vi "NMRFMTCP4.vi"() -> ()   [LabVIEW 2013]
uses:
  <vilib>/Analysis/2dsp.llb/Power Spectrum (DBL).vi
  kleinjan/MKS/Global - Pressure & Flow.vi
  <vilib>/Analysis/NI_AALBase.lvlib
  <vilib>/Analysis/NI_AALPro.lvlib
panel:
  out "Date / Time":string
  in  "Stop Run":bool=TRUE
  out "He readback":bool
  in  "Prompt?":bool
  out "He temp (K)":sgl=2.13326 format="%.3f"
  out "He press (torr)":sgl=33.89 format="%.3f"
  in  "NMR Channel Select":string(combo)="TEQ3560970472.csv"
  out "Color Box":u32(colorbox)=16775210
  out "Measurement":enum16{"TEQ", "POL", "QCV"}(ring)
  in  "IP Address":string="192.168.0.4"
  out "FFT Vrms":dbl[](graph)=[0.003860349127182048, 0.0026408786012199893, 0.0007110928431247576, 0.0002546953194851482, 0.00015606911370408223, 9.557131850537587e-05, 6.115097315115159e-05, 5.7012338680199956e-05, 3.020882234188072e-05, 4.4076193714080254e-05, 2.587519577753813e-05, 1.8713879048394136e-05, 1.6317240401098503e-05, 1.154265718789615e-05, 1.3123955910470731e-05, 1.3368904190798972e-05, 2.1885613497622673e-05, 1.798375515711528e-05, 4.375407331352679e-06, 8.732198758705414e-06, 2.6302534374244283e-06, 3.2949830538442704e-06, 1.1895815050496237e-05, 1.0182966066280883e-05, 1.8847898071173534e-06, 1.3934803392647094e-05, 1.052370134660737e-05, 1.3243501801509567e-05, 8.33538912191352e-06, 9.019609544923987e-06, 8.15332480790813e-06, 1.2373575068285524e-05, 6.708411703327406e-06, 6.22265423944835e-06, 5.068989993909897e-06, 3.0229813974287557e-06, 3.1089525018908967e-06, 5.953693945801889e-06, 6.206631518386126e-06, 6.229207375312059e-06, 4.1144781836691055e-06, 4.354798865838496e-06, 7.172496369868693e-06, 7.0098775910119696e-06, 2.191966447460206e-06, 1.5496079690644168e-06, 4.61696885546102e-06, 3.050901033352866e-06, 4.2174192750427694e-06, 7.930944150085501e-06, 6.689445166261909e-06, 2.1395244143303516e-06, 4.992797769241477e-06, 5.3745245406992406e-06, 6.062617096484538e-07, 8.270129726211426e-06, 3.5956569203627086e-06, 3.008894228477979e-06, 2.398514262112273e-06, 3.4988542677430917e-06, 1.4469323236866402e-06, 3.761661179538815e-06, 3.208518773411313e-06, 1.1187481039417038e-06, 5.7410915598327405e-06, 2.1784164294899814e-06, 3.898449684772871e-06, 3.52083007717426e-06, 1.9374004848225125e-06, 4.891889867434457e-06, 6.02715900907592e-06, 4.437968762435767e-06, 9.263245466394894e-07, 1.8616505810287503e-06, 5.23877964116065e-06, 3.0516904937122464e-06, 1.2800285909118407e-06, 3.507863659114302e-06, 6.239420652579072e-06, 5.998691457241049e-06, 5.312274179144818e-06, 3.3537794541369595e-06, 4.01592999534701e-06, 3.4824037830326406e-06, 3.0526271910251635e-06, 2.0097727604825172e-07, 4.607643528464001e-06, 5.424380631868744e-07, 4.160257383574649e-06, 2.972658642662555e-06, 1.9597322124373752e-06, 1.5255511381117527e-06, 2.103017178478501e-06, 5.198777606068562e-06, 2.9880903247162306e-06, 2.893406927495963e-06, 7.540072348828783e-06, 4.438692918242774e-06, 3.247269316126007e-06, 2.0747730164845625e-06, 6.856536235717e-06, 2.6481781470338664e-06, 3.0193029912273966e-06, 2.408089360787412e-06, 1.5854430464411955e-06, 1.8285871190437193e-06, 5.678656730464855e-06, 1.3784893037679748e-06, 4.116812883085481e-06, 4.819248986093936e-06, 4.5984658016483224e-06, 8.93008614072191e-06, 1.9094683248174202e-06, 9.416405140841326e-07, 5.047384071163484e-06, 3.197206859072784e-06, 1.794238609540721e-06, 3.313919423173037e-06, 2.714293243229963e-06, 3.535772500382675e-06, 3.499416768329835e-06, 4.63435639488753e-06, 5.034221148869452e-06, 1.8865455693025404e-06, 1.7901292369306268e-06, 4.424636665427706e-06, 5.615437490712334e-06, 2.466160580053458e-06, 2.1963153825552336e-06, 1.4846089900612258e-06, 4.302151200697518e-06, 5.254114798762438e-06, 3.1704642311621737e-06, 5.0703036462118136e-06, 1.354955104532314e-06, 3.0453363933660534e-06, 2.2463152825410145e-06, 3.808846738627808e-06, 3.7092372363585685e-06, 1.6325106978788555e-06, 3.2360511524404856e-06, 4.7480841852563215e-06, 5.2505859441000515e-06, 3.2850893327834457e-06, 1.934541747732607e-06, 3.029163168561454e-06, 1.9691995667214222e-06, 3.6405323264696174e-06, 5.056036709880387e-06, 1.919493519278465e-06, 5.595589965036569e-06, 1.852477214655658e-06, 2.8684687433525202e-06, 3.335542196883582e-06, 1.5704926166201195e-06, 3.7962328761918072e-06, 2.6584497284681668e-06, 3.4851642706109724e-06, 6.07788348181537e-06, 2.053548477567382e-06, 9.021564390261138e-07, 2.0277807693204723e-06, 4.32296683764549e-06, 4.064631037560265e-06, 3.8020871322129444e-06, 5.083401813415545e-06, 1.6733656079193586e-06, 1.745150362223994e-06, 8.979218241770401e-07, 1.531740077054345e-06, 5.921042959376128e-06, 2.424206120086413e-06, 6.426437182740756e-06, 5.5924058263776714e-06, 3.5215389749528754e-06, 8.300291245529953e-07, 4.411015274857682e-06, 2.563127166962874e-06, 5.846484935826142e-06, 3.130939375184453e-06, 2.719666304224687e-06, 7.360092224187938e-06, 1.7194250571999971e-06, 1.5443725434450432e-06, 3.822361300685473e-06, 3.923937068239552e-06, 2.89002198233437e-06, 1.614324549229591e-06, 2.999584927529115e-06, 2.060886472403204e-06, 1.3378034874859538e-06, 1.4706542842267576e-06, 3.536883042238073e-06, 7.249143652381299e-06, 1.267328794401466e-06, 1.1086696271129312e-06, 3.927146285844193e-06, 2.3360865908334468e-06, 2.672841677564323e-06, 3.4481594062109245e-06, 1.9525353575254287e-06, 1.9525353575254287e-06, 3.4481594062109245e-06, 2.672841677564323e-06, 2.3360865908334468e-06, 3.927146285844193e-06, 1.1086696271129312e-06, 1.267328794401466e-06, 7.249143652381299e-06, 3.536883042238073e-06, 1.4706542842267576e-06, 1.3378034874859538e-06, 2.060886472403204e-06, 2.999584927529115e-06, 1.614324549229591e-06, 2.89002198233437e-06, 3.923937068239552e-06, 3.822361300685473e-06, 1.5443725434450432e-06, 1.7194250571999971e-06, 7.360092224187938e-06, 2.719666304224687e-06, 3.130939375184453e-06, 5.846484935826142e-06, 2.563127166962874e-06, 4.411015274857682e-06, 8.300291245529953e-07, 3.5215389749528754e-06, 5.5924058263776714e-06, 6.426437182740756e-06, 2.424206120086413e-06, 5.921042959376128e-06, 1.531740077054345e-06, 8.979218241770401e-07, 1.745150362223994e-06, 1.6733656079193586e-06, 5.083401813415545e-06, 3.8020871322129444e-06, 4.064631037560265e-06, 4.32296683764549e-06, 2.0277807693204723e-06, 9.021564390261138e-07, 2.053548477567382e-06, 6.07788348181537e-06, 3.4851642706109724e-06, 2.6584497284681668e-06, 3.7962328761918072e-06, 1.5704926166201195e-06, 3.335542196883582e-06, 2.8684687433525202e-06, 1.852477214655658e-06, 5.595589965036569e-06, 1.919493519278465e-06, 5.056036709880387e-06, 3.6405323264696174e-06, 1.9691995667214222e-06, 3.029163168561454e-06, 1.934541747732607e-06, 3.2850893327834457e-06, 5.2505859441000515e-06, 4.7480841852563215e-06, 3.2360511524404856e-06, 1.6325106978788555e-06, 3.7092372363585685e-06, 3.808846738627808e-06, 2.2463152825410145e-06, 3.0453363933660534e-06, 1.354955104532314e-06, 5.0703036462118136e-06, 3.1704642311621737e-06, 5.254114798762438e-06, 4.302151200697518e-06, 1.4846089900612258e-06, 2.1963153825552336e-06, 2.466160580053458e-06, 5.615437490712334e-06, 4.424636665427706e-06, 1.7901292369306268e-06, 1.8865455693025404e-06, 5.034221148869452e-06, 4.63435639488753e-06, 3.499416768329835e-06, 3.535772500382675e-06, 2.714293243229963e-06, 3.313919423173037e-06, 1.794238609540721e-06, 3.197206859072784e-06, 5.047384071163484e-06, 9.416405140841326e-07, 1.9094683248174202e-06, 8.93008614072191e-06, 4.5984658016483224e-06, 4.819248986093936e-06, 4.116812883085481e-06, 1.3784893037679748e-06, 5.678656730464855e-06, 1.8285871190437193e-06, 1.5854430464411955e-06, 2.408089360787412e-06, 3.0193029912273966e-06, 2.6481781470338664e-06, 6.856536235717e-06, 2.0747730164845625e-06, 3.247269316126007e-06, 4.438692918242774e-06, 7.540072348828783e-06, 2.893406927495963e-06, 2.9880903247162306e-06, 5.198777606068562e-06, 2.103017178478501e-06, 1.5255511381117527e-06, 1.9597322124373752e-06, 2.972658642662555e-06, 4.160257383574649e-06, 5.424380631868744e-07, 4.607643528464001e-06, 2.0097727604825172e-07, 3.0526271910251635e-06, 3.4824037830326406e-06, 4.01592999534701e-06, 3.3537794541369595e-06, 5.312274179144818e-06, 5.998691457241049e-06, 6.239420652579072e-06, 3.507863659114302e-06, 1.2800285909118407e-06, 3.0516904937122464e-06, 5.23877964116065e-06, 1.8616505810287503e-06, 9.263245466394894e-07, 4.437968762435767e-06, 6.02715900907592e-06, 4.891889867434457e-06, 1.9374004848225125e-06, 3.52083007717426e-06, 3.898449684772871e-06, 2.1784164294899814e-06, 5.7410915598327405e-06, 1.1187481039417038e-06, 3.208518773411313e-06, 3.761661179538815e-06, 1.4469323236866402e-06, 3.4988542677430917e-06, 2.398514262112273e-06, 3.008894228477979e-06, 3.5956569203627086e-06, 8.270129726211426e-06, 6.062617096484538e-07, 5.3745245406992406e-06, 4.992797769241477e-06, 2.1395244143303516e-06, 6.689445166261909e-06, 7.930944150085501e-06, 4.2174192750427694e-06, 3.050901033352866e-06, 4.61696885546102e-06, 1.5496079690644168e-06, 2.191966447460206e-06, 7.0098775910119696e-06, 7.172496369868693e-06, 4.354798865838496e-06, 4.1144781836691055e-06, 6.229207375312059e-06, 6.206631518386126e-06, 5.953693945801889e-06, 3.1089525018908967e-06, 3.0229813974287557e-06, 5.068989993909897e-06, 6.22265423944835e-06, 6.708411703327406e-06, 1.2373575068285524e-05, 8.15332480790813e-06, 9.019609544923987e-06, 8.33538912191352e-06, 1.3243501801509567e-05, 1.052370134660737e-05, 1.3934803392647094e-05, 1.8847898071173534e-06, 1.0182966066280883e-05, 1.1895815050496237e-05, 3.2949830538442704e-06, 2.6302534374244283e-06, 8.732198758705414e-06, 4.375407331352679e-06, 1.798375515711528e-05, 2.1885613497622673e-05, 1.3368904190798972e-05, 1.3123955910470731e-05, 1.154265718789615e-05, 1.6317240401098503e-05, 1.8713879048394136e-05, 2.587519577753813e-05, 4.4076193714080254e-05, 3.020882234188072e-05, 5.7012338680199956e-05, 6.115097315115159e-05, 9.557131850537587e-05, 0.00015606911370408223, 0.0002546953194851482, 0.0007110928431247576, 0.0026408786012199893]
  out "Raw NMR Graph / Ave":cluster{dbl, "Step Width (MHz)":dbl, dbl[][]}(graph)={212.6, "Step Width (MHz)"=0.002, [[0.0121, 0.0117, 0.0117, 0.0117, 0.0114, 0.0113, 0.0113, 0.0111, 0.0111, 0.011, 0.011, 0.0108, 0.0107, 0.0105, 0.0105, 0.0104, 0.0099, 0.0099, 0.0098, 0.0096, 0.0096, 0.0095, 0.0095, 0.0093, 0.0093, 0.0092, 0.0089, 0.0089, 0.0087, 0.0085, 0.0084, 0.0084, 0.0081, 0.0081, 0.0079, 0.0079, 0.0078, 0.0076, 0.0076, 0.0076, 0.0075, 0.0073, 0.0073, 0.0072, 0.0072, 0.007, 0.0069, 0.0067, 0.0067, 0.0066, 0.0064, 0.0061, 0.0063, 0.0061, 0.006, 0.006, 0.0056, 0.0056, 0.0055, 0.0053, 0.0053, 0.0052, 0.0052, 0.005, 0.005, 0.0049, 0.0049, 0.0047, 0.0046, 0.0046, 0.0044, 0.0046, 0.0044, 0.0044, 0.0041, 0.0041, 0.004, 0.0038, 0.0038, 0.0038, 0.0035, 0.0035, 0.0035, 0.0034, 0.0034, 0.0034, 0.0032, 0.0031, 0.0029, 0.0029, 0.0029, 0.0029, 0.0027, 0.0026, 0.0026, 0.0026, 0.0024, 0.0024, 0.0023, 0.0021, 0.0021, 0.0021, 0.002, 0.002, 0.002, 0.0018, 0.0018, 0.0017, 0.0017, 0.0015, 0.0015, 0.0015, 0.0015, 0.0014, 0.0014, 0.0014, 0.0012, 0.0012, 0.0012, 0.0011, 0.0011, 0.0011, 0.0011, 0.0009, 0.0009, 0.0009, 0.0009, 0.0008, 0.0008, 0.0008, 0.0006, 0.0005, 0.0005, 0.0005, 0.0003, 0.0005, 0.0005, 0.0003, 0.0003, 0.0003, 0.0002, 0.0002, 0.0002, 0.0002, 0.0002, -0.0, -0.0, -0.0, -0.0, -0.0, -0.0, -0.0, -0.0, -0.0002, -0.0, -0.0, -0.0, -0.0002, -0.0, -0.0, -0.0, -0.0, -0.0, -0.0, -0.0, -0.0, -0.0, -0.0002, -0.0002, -0.0002, -0.0002, -0.0002, -0.0002, -0.0002, -0.0002, -0.0002, -0.0003, -0.0002, -0.0003, -0.0003, -0.0003, -0.0003, -0.0005, -0.0003, -0.0003, -0.0003, -0.0003, -0.0003, -0.0003, -0.0003, -0.0003, -0.0003, -0.0003, -0.0003, -0.0005, -0.0003, -0.0005, -0.0005, -0.0006, -0.0003, -0.0003, -0.0003, -0.0003, -0.0003, -0.0003, -0.0003, -0.0002, -0.0003, -0.0003, -0.0003, -0.0002, -0.0003, -0.0002, -0.0002, -0.0002, -0.0, -0.0, -0.0, -0.0002, -0.0002, -0.0, -0.0, -0.0, -0.0, -0.0, -0.0, -0.0, -0.0, -0.0, -0.0, -0.0, -0.0, -0.0, -0.0, -0.0, 0.0002, -0.0, 0.0002, -0.0, 0.0002, 0.0002, 0.0003, 0.0002, 0.0002, 0.0003, 0.0003, 0.0005, 0.0003, 0.0005, 0.0005, 0.0005, 0.0006, 0.0006, 0.0008, 0.0008, 0.0009, 0.0008, 0.0008, 0.0009, 0.0008, 0.0009, 0.0009, 0.0008, 0.0011, 0.0009, 0.0011, 0.0012, 0.0012, 0.0014, 0.0014, 0.0014, 0.0015, 0.0015, 0.0015, 0.0017, 0.0017, 0.0017, 0.0018, 0.0018, 0.0018, 0.0018, 0.0018, 0.0018, 0.002, 0.002, 0.0021, 0.0023, 0.0023, 0.0023, 0.0023, 0.0024, 0.0026, 0.0026, 0.0027, 0.0027, 0.0029, 0.0029, 0.0029, 0.0031, 0.0031, 0.0031, 0.0031, 0.0034, 0.0034, 0.0035, 0.0035, 0.0035, 0.0037, 0.0037, 0.0038, 0.0038, 0.0038, 0.004, 0.004, 0.0041, 0.0041, 0.0043, 0.0044, 0.0044, 0.0046, 0.0047, 0.0047, 0.0049, 0.0049, 0.0052, 0.0052, 0.005, 0.0052, 0.0053, 0.0053, 0.0055, 0.0055, 0.0058, 0.0058, 0.0058, 0.0058, 0.006, 0.0061, 0.0061, 0.0063, 0.0064, 0.0066, 0.0066, 0.0066, 0.0067, 0.0069, 0.007, 0.0072, 0.0072, 0.0073, 0.0075, 0.0075, 0.0076, 0.0076, 0.0078, 0.0078, 0.0079, 0.0081, 0.0082, 0.0084, 0.0084, 0.0085, 0.0085, 0.0087, 0.0089, 0.0089, 0.0089, 0.0092, 0.0093, 0.0093, 0.0095, 0.0096, 0.0096, 0.0096, 0.0099, 0.0099, 0.0101, 0.0101, 0.0102, 0.0104, 0.0105, 0.0105, 0.0107, 0.0108, 0.011, 0.011, 0.011, 0.0111, 0.0113, 0.0114, 0.0116, 0.0116, 0.0117, 0.0119, 0.0119, 0.0121, 0.0122, 0.0124, 0.0125, 0.0125, 0.0127], [0.0, 0.0, 0.0, 0.0, 0.0, 0.0, 0.0, 0.0, 0.0, 0.0, 0.0, 0.0, 0.0, 0.0, 0.0, 0.0, 0.0, 0.0, 0.0, 0.0, 0.0, 0.0, 0.0, 0.0, 0.0, 0.0, 0.0, 0.0, 0.0, 0.0, 0.0, 0.0, 0.0, 0.0, 0.0, 0.0, 0.0, 0.0, 0.0, 0.0, 0.0, 0.0, 0.0, 0.0, 0.0, 0.0, 0.0, 0.0, 0.0, 0.0, 0.0, 0.0, 0.0, 0.0, 0.0, 0.0, 0.0, 0.0, 0.0, 0.0, 0.0, 0.0, 0.0, 0.0, 0.0, 0.0, 0.0, 0.0, 0.0, 0.0, 0.0, 0.0, 0.0, 0.0, 0.0, 0.0, 0.0, 0.0, 0.0, 0.0, 0.0, 0.0, 0.0, 0.0, 0.0, 0.0, 0.0, 0.0, 0.0, 0.0, 0.0, 0.0, 0.0, 0.0, 0.0, 0.0, 0.0, 0.0, 0.0, 0.0, 0.0, 0.0, 0.0, 0.0, 0.0, 0.0, 0.0, 0.0, 0.0, 0.0, 0.0, 0.0, 0.0, 0.0, 0.0, 0.0, 0.0, 0.0, 0.0, 0.0, 0.0, 0.0, 0.0, 0.0, 0.0, 0.0, 0.0, 0.0, 0.0, 0.0, 0.0, 0.0, 0.0, 0.0, 0.0, 0.0, 0.0, 0.0, 0.0, 0.0, 0.0, 0.0, 0.0, 0.0, 0.0, 0.0, 0.0, 0.0, 0.0, 0.0, 0.0, 0.0, 0.0, 0.0, 0.0, 0.0, 0.0, 0.0, 0.0, 0.0, 0.0, 0.0, 0.0, 0.0, 0.0, 0.0, 0.0, 0.0, 0.0, 0.0, 0.0, 0.0, 0.0, 0.0, 0.0, 0.0, 0.0, 0.0, 0.0, 0.0, 0.0, 0.0, 0.0, 0.0, 0.0, 0.0, 0.0, 0.0, 0.0, 0.0, 0.0, 0.0, 0.0, 0.0, 0.0, 0.0, 0.0, 0.0, 0.0, 0.0, 0.0, 0.0, 0.0, 0.0, 0.0, 0.0, 0.0, 0.0, 0.0, 0.0, 0.0, 0.0, 0.0, 0.0, 0.0, 0.0, 0.0, 0.0, 0.0, 0.0, 0.0, 0.0, 0.0, 0.0, 0.0, 0.0, 0.0, 0.0, 0.0, 0.0, 0.0, 0.0, 0.0, 0.0, 0.0, 0.0, 0.0, 0.0, 0.0, 0.0, 0.0, 0.0, 0.0, 0.0, 0.0, 0.0, 0.0, 0.0, 0.0, 0.0, 0.0, 0.0, 0.0, 0.0, 0.0, 0.0, 0.0, 0.0, 0.0, 0.0, 0.0, 0.0, 0.0, 0.0, 0.0, 0.0, 0.0, 0.0, 0.0, 0.0, 0.0, 0.0, 0.0, 0.0, 0.0, 0.0, 0.0, 0.0, 0.0, 0.0, 0.0, 0.0, 0.0, 0.0, 0.0, 0.0, 0.0, 0.0, 0.0, 0.0, 0.0, 0.0, 0.0, 0.0, 0.0, 0.0, 0.0, 0.0, 0.0, 0.0, 0.0, 0.0, 0.0, 0.0, 0.0, 0.0, 0.0, 0.0, 0.0, 0.0, 0.0, 0.0, 0.0, 0.0, 0.0, 0.0, 0.0, 0.0, 0.0, 0.0, 0.0, 0.0, 0.0, 0.0, 0.0, 0.0, 0.0, 0.0, 0.0, 0.0, 0.0, 0.0, 0.0, 0.0, 0.0, 0.0, 0.0, 0.0, 0.0, 0.0, 0.0, 0.0, 0.0, 0.0, 0.0, 0.0, 0.0, 0.0, 0.0, 0.0, 0.0, 0.0, 0.0, 0.0, 0.0, 0.0, 0.0, 0.0, 0.0, 0.0, 0.0, 0.0, 0.0, 0.0, 0.0, 0.0, 0.0, 0.0, 0.0, 0.0, 0.0, 0.0, 0.0, 0.0, 0.0, 0.0, 0.0, 0.0, 0.0, 0.0, 0.0, 0.0, 0.0, 0.0, 0.0, 0.0, 0.0, 0.0, 0.0, 0.0, 0.0, 0.0, 0.0, 0.0, 0.0, 0.0, 0.0, 0.0, 0.0, 0.0, 0.0]]}
  in  "GPIB Addr (28)":refnum<visa-resource-name>="GPIB1::28::INSTR"
  out "Pedestal (V)":dbl=0.006282083333333333 format="%_2g"
  in  "Open Global Panel":bool=TRUE
  out "Peak center (MHz)":sgl=213.38817 format="%.3f"
  out "Telnet error out":errorcluster
  out "+3.3V supply":dbl=3.265 format="%_4g"
  out "Temp (C)":dbl=27.5 format="%_4g"
  out "RF OK":bool=TRUE
  out "Peak area (V-MHz)":sgl=-1.9332666 format="%.5f"
  out "# Good Spectra":i32=1000
  out "Pedestal OK":bool=TRUE
  out "Sweep #":i32=6
  out "1st Sweep":bool
  out "ADC volts OK":bool=TRUE
  out "Peak Height Distribution":cluster{"Y":dbl[], "Y":dbl[]}[](graph)=[{"Y"=[0.008008147916666668, 0.008026943750000001, 0.008045739583333334, 0.008064535416666668, 0.00808333125, 0.008102127083333334, 0.008120922916666667, 0.00813971875, 0.008158514583333333, 0.008177310416666667, 0.00819610625, 0.008214902083333335, 0.008233697916666668, 0.008252493750000001, 0.008271289583333334, 0.008290085416666667, 0.00830888125, 0.008327677083333334, 0.008346472916666667, 0.00836526875, 0.008384064583333333, 0.008402860416666666, 0.008421656250000001, 0.008440452083333334, 0.008459247916666668, 0.00847804375, 0.008496839583333334, 0.008515635416666667, 0.00853443125, 0.008553227083333333, 0.008572022916666667, 0.00859081875, 0.008609614583333333, 0.008628410416666668, 0.008647206250000001, 0.008666002083333334, 0.008684797916666667, 0.00870359375, 0.008722389583333334, 0.008741185416666667, 0.00875998125, 0.008778777083333333, 0.008797572916666666, 0.00881636875, 0.008835164583333333, 0.008853960416666667, 0.00887275625, 0.008891552083333334, 0.008910347916666667, 0.00892914375, 0.008947939583333333, 0.008966735416666666, 0.00898553125, 0.009004327083333333, 0.009023122916666666, 0.009041918749999999, 0.009060714583333334, 0.009079510416666667, 0.00909830625, 0.009117102083333333, 0.009135897916666667, 0.00915469375, 0.009173489583333333, 0.009192285416666666, 0.00921108125, 0.009229877083333332, 0.009248672916666666, 0.00926746875, 0.009286264583333334, 0.009305060416666667, 0.00932385625, 0.009342652083333333, 0.009361447916666666, 0.00938024375, 0.009399039583333333, 0.009417835416666666, 0.009436631249999999, 0.009455427083333332, 0.009474222916666667, 0.00949301875, 0.009511814583333333, 0.009530610416666667, 0.00954940625, 0.009568202083333333, 0.009586997916666666, 0.00960579375, 0.009624589583333332, 0.009643385416666666, 0.009662181249999999, 0.009680977083333334, 0.009699772916666667, 0.00971856875, 0.009737364583333333, 0.009756160416666666, 0.00977495625, 0.009793752083333333, 0.009812547916666666, 0.009831343749999999, 0.009850139583333332, 0.009868935416666665], "Y"=[1.0, 0.0, 0.0, 1.0, 1.0, 0.0, 2.0, 1.0, 1.0, 1.0, 2.0, 2.0, 4.0, 2.0, 2.0, 3.0, 3.0, 3.0, 4.0, 3.0, 5.0, 6.0, 4.0, 4.0, 7.0, 3.0, 10.0, 5.0, 10.0, 7.0, 9.0, 8.0, 14.0, 12.0, 9.0, 16.0, 10.0, 17.0, 13.0, 14.0, 12.0, 10.0, 24.0, 21.0, 12.0, 18.0, 16.0, 23.0, 22.0, 15.0, 16.0, 19.0, 16.0, 19.0, 14.0, 17.0, 23.0, 22.0, 22.0, 24.0, 23.0, 22.0, 17.0, 25.0, 18.0, 23.0, 20.0, 14.0, 14.0, 10.0, 18.0, 20.0, 10.0, 20.0, 16.0, 10.0, 13.0, 14.0, 12.0, 11.0, 15.0, 10.0, 11.0, 7.0, 6.0, 9.0, 0.0, 8.0, 3.0, 3.0, 4.0, 3.0, 3.0, 1.0, 0.0, 0.0, 0.0, 1.0, 1.0, 1.0]}]
  out "S/N":dbl=26.093843753781734 format="%_3g"
  out "Peak mean (V)":dbl=0.009030414166666665 format="%_4g"
  out "Pedestal Diff (V)":sgl=0.0009175 format="%.3f"
  out "Peak amp (V)":sgl=0.0064179166 format="%.3f"
  out "SMT error out":errorcluster
  out "Peak RMS (mV)":dbl=0.3460745090633841 format="%.3f"
  # "E1039 NMR Panel"
  # "Results"
  # "A\nv\ne\nr\na\ng\ne\ns"
  # "S\nw\ne\ne\np"
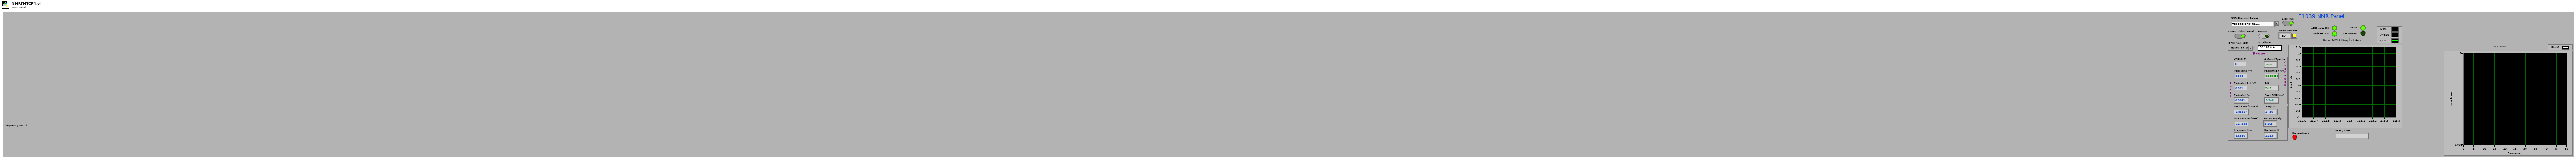
[diagram p1: front panel]
types:
  T1 = enum32{"Invalid", "Standard", "Closed", "Hidden", "Minimized", "Maximized"}
  T2 = enum32{"Bad", "Idle", "Run top level", "Running"}
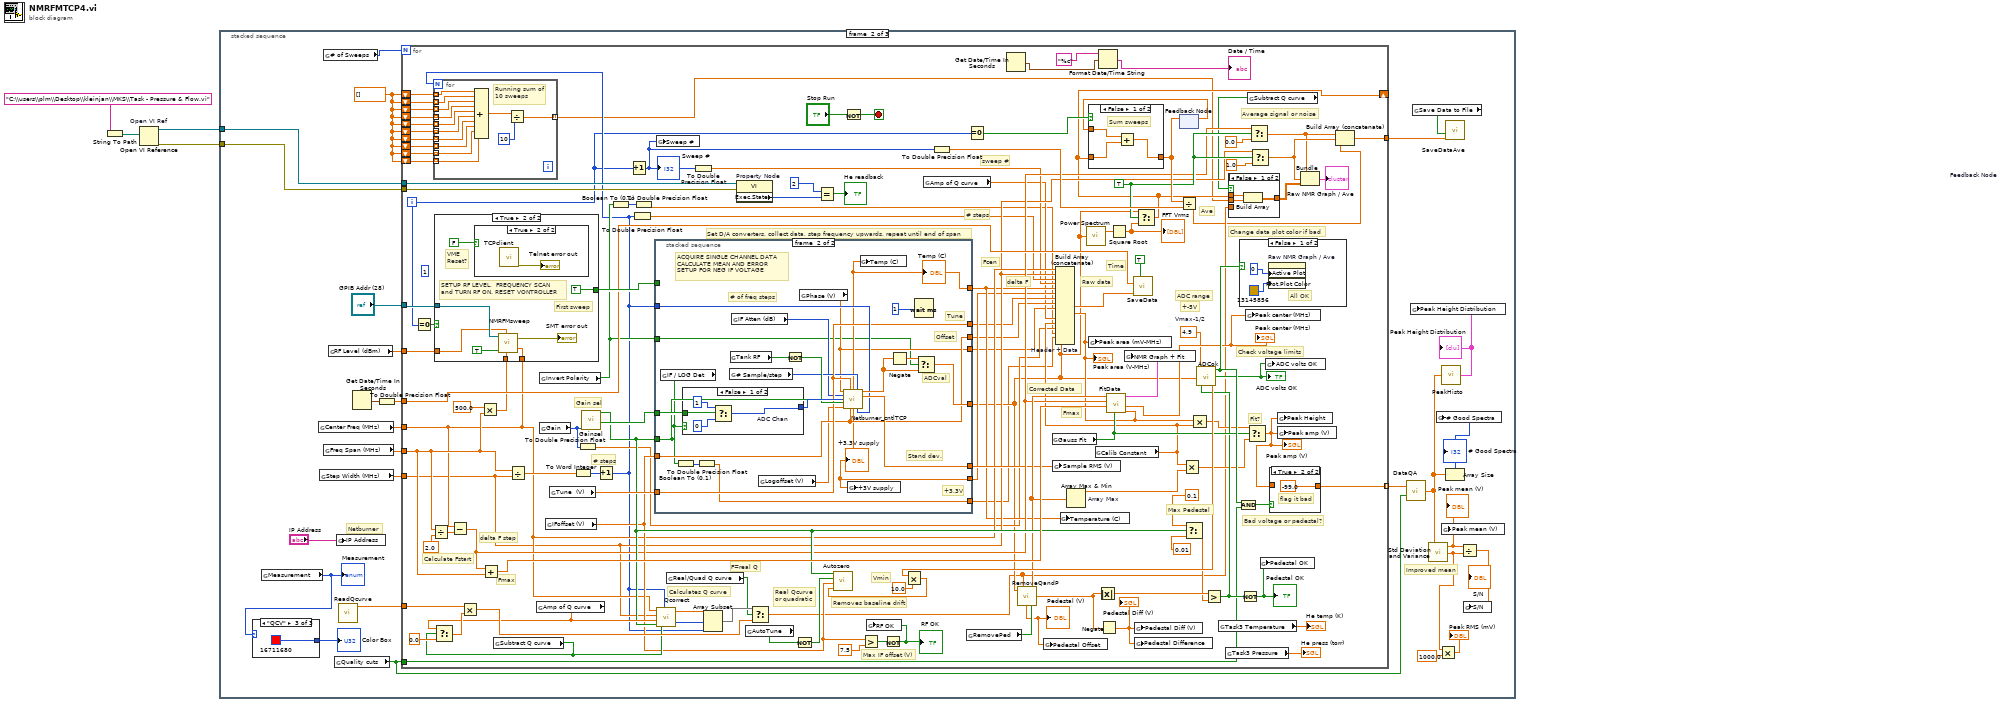
[diagram p0: block diagram]
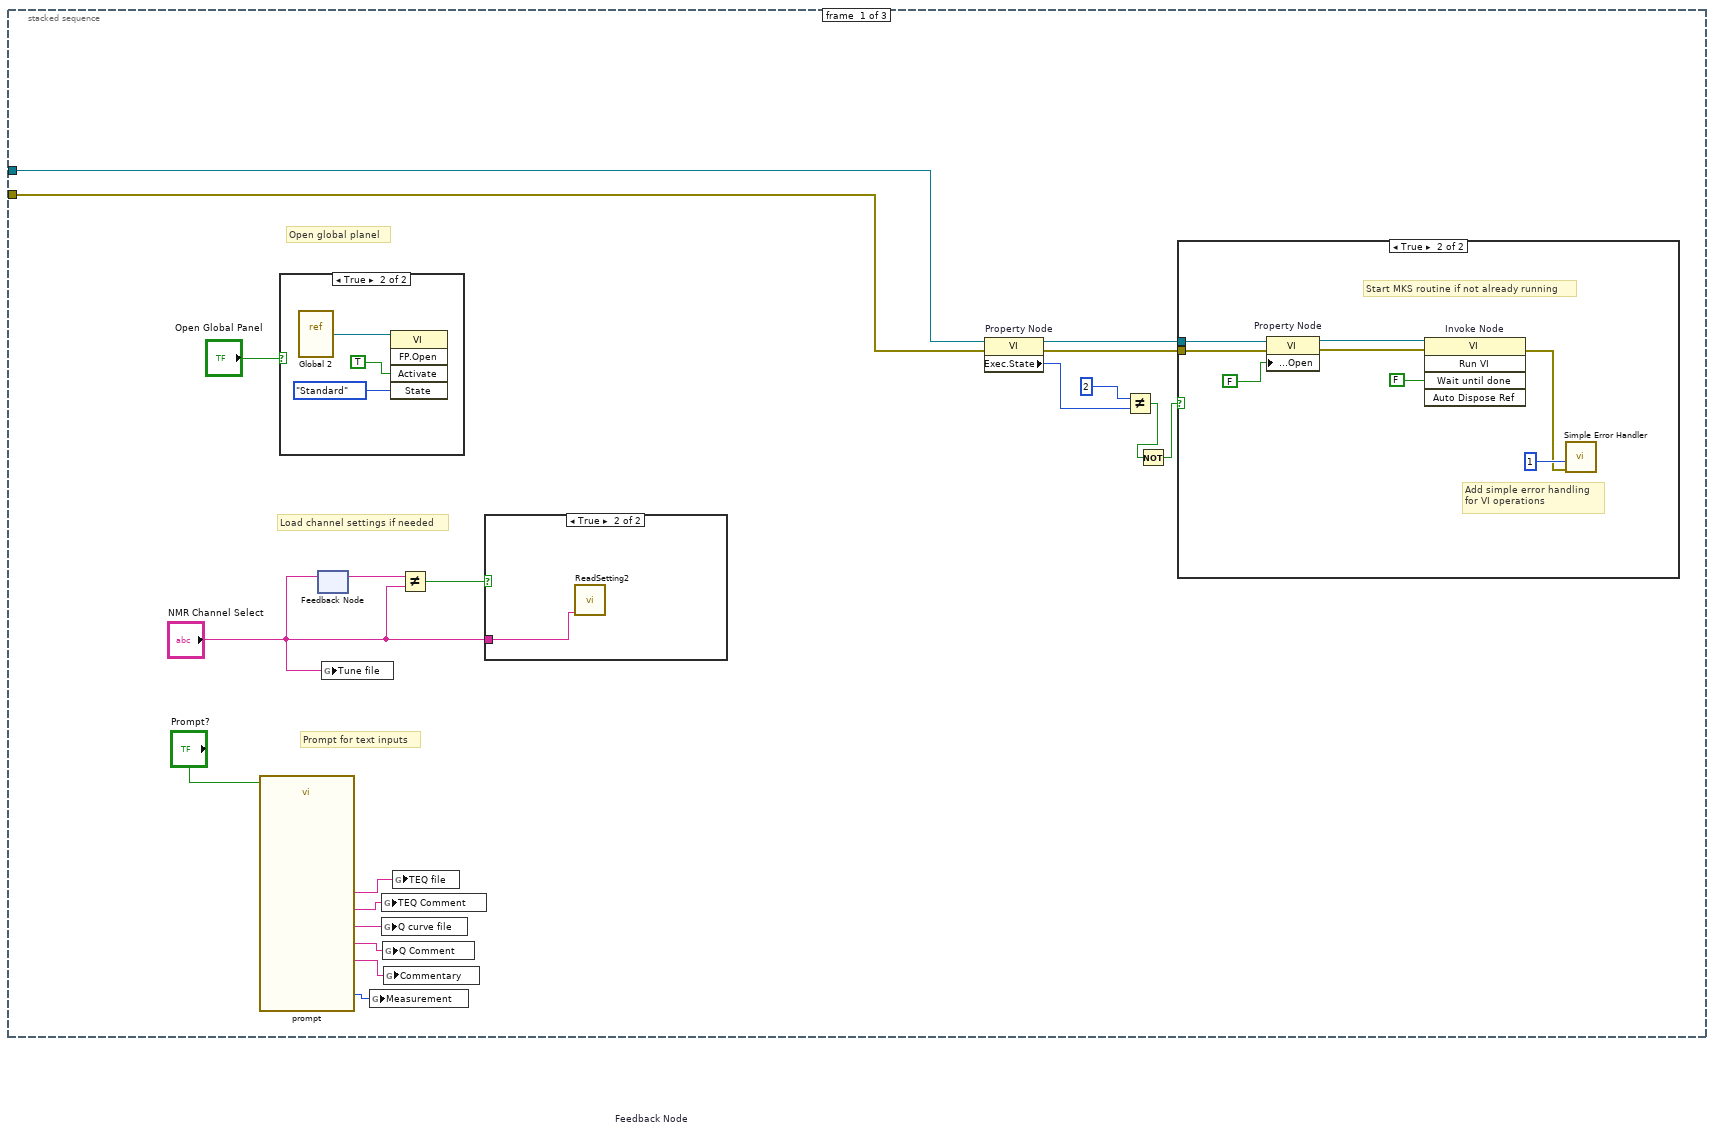
[diagram p2: hidden frame]
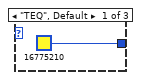
[diagram p6: hidden frame]
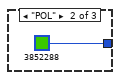
[diagram p7: hidden frame]
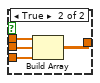
[diagram p8: hidden frame]
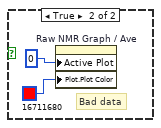
[diagram p10: hidden frame]
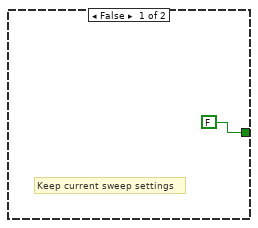
[diagram p12: hidden frame]
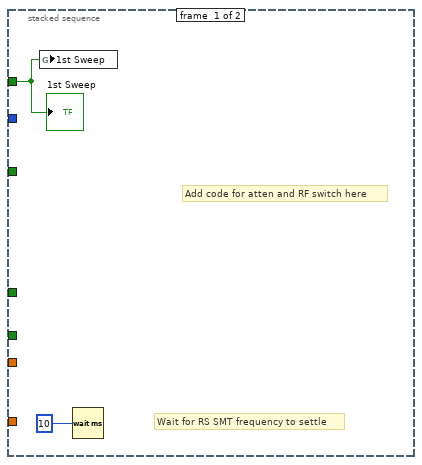
[diagram p14: hidden frame]
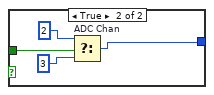
[diagram p15: hidden frame]
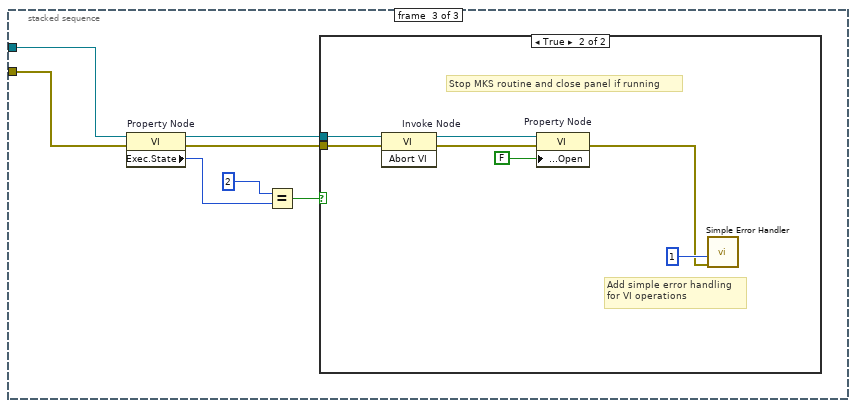
[diagram p16: hidden frame]
diagram:
  n1 = String To Path(string="C:\\users\\plm\\Desktop\\kleinjan\\MKS\\Task - Pressure & Flow.vi") -> (path=w4:path)
  n2 = Open VI Reference "Open VI Ref"(vi path=w4) -> (vi reference=w1:refnum<vi>, error out=w2:errorcluster)  [unwired: 5 in]
  n3 = stacked-sequence {
    tunnel: w1 -> [w8 w38 w266]
    tunnel: w2 -> [w7 w37 w265]
    frame #0 {
      # "Prompt for text inputs"
      # "Load channel settings if needed"
      # "Open global planel"
      n4 = call "prompt.vi"("Enable"="Prompt?") -> ("Measurement"=w21:enum16{"TEQ", "POL", "QCV"}, "Run comment"=w20:string, "Q curve comment"=w19:string, "Q curve file"=w18:string, "TE Comment"=w17:string, "TE peak file"=w16:string)  [unwired: 11 in, 2 out]
      n5 = case shown="True" "Open Global Panel" {
        frame False {
        }
        frame True {
          n6 = vi-ref "Global 2.vi"() -> (w35:refnum<vi>)
          n7 = invoke class="VI" method="FP.Open"(reference=w35, "Activate"=TRUE, "State"=T1."Standard") -> ()  [unwired: 2 in, 5 out]
        }
      }
      n8 = feedback #1 "Feedback Node"() -> (w15:string)  [unwired: 1 in]
      n9 = feedback-in #1("NMR Channel Select") -> ()
      n10 = global write "Global 2.vi" "Tune file"("NMR Channel Select") -> ()
      n11 = global write "Global 2.vi" "Measurement"(w21) -> ()
      n12 = global write "Global 2.vi" "TEQ Comment"(w17) -> ()
      n13 = global write "Global 2.vi" "Q curve file"(w18) -> ()
      n14 = global write "Global 2.vi" "Q Comment"(w19) -> ()
      n15 = global write "Global 2.vi" "Commentary"(w20) -> ()
      n16 = global write "Global 2.vi" "TEQ file"(w16) -> ()
      n17 = Not Equal?(x=w15, y="NMR Channel Select") -> (x != y?=w14:bool)
      n18 = case shown="True" w14 {
        tunnel: "NMR Channel Select" -> [_ w32]
        frame False {
        }
        frame True {
          n19 = call "ReadSetting2.vi"("Data Filename"=w32) -> ()  [unwired: 2 in, 1 out]
        }
      }
      n20 = property on="Property Node" class="VI"(reference=w8, error in=w7) -> (reference out=w10:refnum<vi>, error out=w9:errorcluster, "Exec.State"=w11:T2)
      n21 = Not Equal?(x=2, y=w11) -> (x != y?=w6:bool)
      n22 = Not(x=w6) -> (.not. x?=w5:bool)
      n23 = case shown="True" w5 {
        tunnel: w10 -> [_ w28]
        tunnel: w9 -> [_ w27]
        frame False {
        }
        frame True {
          # "Start MKS routine if not already running"
          # "Add simple error handling\nfor VI operations"
          n24 = property on="Property Node" class="VI"(reference=w28, error in=w27, "Front Panel Window:Open"=FALSE ("Front Panel.Open")) -> (reference out=w26:refnum<vi>, error out=w25:errorcluster)
          n25 = invoke on="Invoke Node" class="VI" method="Run VI"(reference=w26, error in=w25, "Wait until done"=FALSE) -> (error out=w29:errorcluster)  [unwired: 2 in, 4 out]
          n26 = call <vilib>:"Simple Error Handler.vi"("type of dialog (OK msg:1)"=1, "error in (no error)"=w29) -> ()  [unwired: 3 in, 5 out]
        }
      }
    }
    frame #1 {
      w36 = dbl[] []
      # "Netburner"
      # "Improved mean"
      n27 = global read "Global 2.vi" "Measurement"() -> (w40:enum16{"TEQ", "POL", "QCV"})
      "Measurement" <- w40
      n28 = case shown="\"QCV\"" w40 {
        tunnel: [u32 16775210 ("Color Box 2") u32 3852288 ("Color Box 2") u32 16711680 ("Color Box 2")] -> w39
        frame "TEQ", Default {
        }
        frame "POL" {
        }
        frame "QCV" {
        }
      }
      "Color Box" <- w39
      n29 = global read "Global 2.vi" "Center Freq (MHz)"() -> (w57:dbl)
      n30 = global read "Global 2.vi" "Step Width (MHz)"() -> (w55:dbl)
      n31 = global read "Global 2.vi" "# of Sweeps"() -> (w59:i32)
      n32 = global read "Global 2.vi" "Freq Span (MHz)"() -> (w56:dbl)
      n33 = global read "Global 2.vi" "RF Level (dBm)"() -> (w58:dbl)
      n34 = global read "Global 2.vi" "Quality cuts"() -> (w54:bool)
      n35 = global write "Global 2.vi" "IP Address"("IP Address") -> ()
      n36 = call "ReadQcurve.vi"() -> ("Array"=w45:dbl[])  [unwired: 2 in]
      n37 = Get Date/Time In Seconds() -> (seconds since 1Jan1904=w60:timestamp)
      n38 = To Double Precision Float(number=w60) -> (double precision float=w46:dbl)
      n39 = for {
        N: w59 -> [_]
        tunnel: [w183] -> w62 mode=indexing
        tunnel: w54 -> [w145]
        tunnel: w57 -> [w118]
        tunnel: w56 -> [w130]
        tunnel: w55 -> [w117]
        tunnel: "GPIB Addr (28)" -> [w179]
        tunnel: w58 -> [w178]
        tunnel: w46 -> [w177]
        tunnel: w45 -> [w170]
        tunnel: [w135] -> w48
        tunnel: w38 -> [w91]
        tunnel: w37 -> [w90]
        shift-right: [w82] -> _
        shift-left: w36 -> [w81]
        shift-left: w36 -> [w72]
        shift-left: w36 -> [w80]
        shift-left: w36 -> [w79]
        shift-left: w36 -> [w78]
        shift-left: w36 -> [w77]
        shift-left: w36 -> [w76]
        shift-left: w36 -> [w75]
        shift-left: w36 -> [w74]
        shift-left: w36 -> [w73]
        i -> [w70]
        stop <- w88 stop-if-true
        (unwired) 1
        w123 = TRUE
        w140 = 4.9  # Vmax-1/2
        # "Average signal or noise"
        # "Check voltage limits"
        # "Ave"
        # "Max Pedestal"
        # "Gain sel"
        # "F=real Q"
        # "Real Qcurve\nor quadratic"
        # "+-5V"
        # "Change data plot color if bad"
        # "Max IF offset (V)"
        # "Fmax"
        # "Fit?"
        # "Fmax"
        # "Time"
        # "Vmin"
        # "Raw data"
        # "Corrected Data"
        # "Fcen"
        # "delta F"
        # "# steps"
        # "ADC range"
        # "sweep #"
        # "Set D/A converters, collect data, step frequency upwards, repeat until end of span"
        # "Calculates Q curve"
        # "Removes baseline drift"
        # "Bad voltage or pedestal?"
        # "# steps"
        # "Calculate Fstart"
        # "delta F step"
        n40 = Equal To 0?(x=w70) -> (x = 0?=w185:bool)
        n41 = Divide(x=w130, y=sgl 2.0) -> (x/y=w189:dbl)
        n42 = Subtract(x=w118, y=w189) -> (x-y=w121:dbl)
        n43 = Multiply(x=500.0, y=w130) -> (x*y=w129:dbl)
        n44 = case shown="True" w185 {
          tunnel: w118 -> [_ w229]
          tunnel: w129 -> [_ w230]
          tunnel: [FALSE TRUE] -> w184
          tunnel: w179 -> [_ w226]
          tunnel: w178 -> [_ w225]
          frame False {
            # "Keep current sweep settings"
          }
          frame True {
            # "VME\nReset?"
            # "First sweep"
            # "SETUP RF LEVEL,  FREQUENCY SCAN\nand TURN RF ON. RESET VONTROLLER"
            n45 = case shown="True" FALSE {
              frame False {
              }
              frame True {
                n46 = call "TCPclient.vi"() -> ("Telnet error"=→"Telnet error out":errorcluster)  [unwired: 4 in, 3 out]
              }
            }
            n47 = call "NMRFMsweep.vi"("Center Freq (MHz)"=w229, "Freq Span (kHz)"=w230, "RF Level (dBm)"=w225, "Program"=TRUE, "GPIB Addr (28)"=w226) -> ("error out"=→"SMT error out":errorcluster)  [unwired: 2 in]
          }
        }
        n48 = Add(x=w121, y=w130) -> (x+y=w174:dbl)
        n49 = global read "Global 2.vi" "Subtract Q curve"() -> (w161:bool)
        n50 = Divide(x=w130, y=w117) -> (x/y=w191:dbl)
        n51 = global read "Global 2.vi" "Amp of Q curve"() -> (w162:dbl)
        n52 = Select(t=w162, s=w161, f=0.0) -> (s? t:f=w167:dbl)
        n53 = Multiply(x=w170, y=w167) -> (x*y=w169:dbl[])
        n54 = global read "Global 2.vi" "Invert Polarity"() -> (w99:bool)
        n55 = global read "Global 2.vi" "Gain"() -> (w104:enum16{"LOW", "HI", "MAX"})
        n56 = global read "Global 2.vi" "IFoffset (V)"() -> (w134:dbl)
        n57 = global read "Global 2.vi" "Tune  (V)"() -> (w163:dbl)
        n58 = To Word Integer(number=w191) -> (16bit integer=w188:i16)
        n59 = To Double Precision Float(number=w104) -> (double precision float=w103:dbl)
        n60 = call "Gainsel.vi"("Gain"=w104) -> ("LO"=w137:bool, "MAX"=w136:bool)  [unwired: 1 out]
        n61 = Increment(x=w188) -> (x+1=w71:i16)
        n62 = for {
          N: w71 -> [_]
          tunnel: w81 -> [w195] mode=indexing
          tunnel: w80 -> [w203] mode=indexing
          tunnel: w79 -> [w202] mode=indexing
          tunnel: w78 -> [w201] mode=indexing
          tunnel: w77 -> [w200] mode=indexing
          tunnel: w76 -> [w199] mode=indexing
          tunnel: w75 -> [w198] mode=indexing
          tunnel: w74 -> [w197] mode=indexing
          tunnel: w73 -> [w196] mode=indexing
          tunnel: w72 -> [w204] mode=indexing
          tunnel: [w192] -> w69 mode=indexing
          # "Running sum of 10 sweeps"
          n63 = Compound Arithmetic op=ADD(w195, w204, w203, w202, w201, w200, w199, w198, w197, w196) -> (w193:dbl)
          n64 = Divide(x=w193, y=10) -> (x/y=w192:dbl)
        }
        n65 = Boolean To (0,1)(Boolean=w99) -> (0, 1=w100:i16)
        n66 = Increment(x=w70) -> (x+1=w143:i32)
        "Sweep #" <- w143
        n67 = To Double Precision Float(number=w71) -> (double precision float=w116:dbl)
        n68 = To Double Precision Float(number=w100) -> (double precision float=w98:dbl)
        n69 = stacked-sequence {
          tunnel: [_ w251] -> w119
          tunnel: [_ w255] -> w102
          tunnel: w71 -> [_ w249]
          tunnel: w134 -> [_ w246]
          tunnel: w137 -> [_ w253]
          tunnel: w184 -> [w232 _]
          tunnel: w163 -> [_ w247]
          tunnel: [_ w240] -> w114
          tunnel: [_ w239] -> w113
          tunnel: [_ w247] -> w112
          tunnel: [_ w246] -> w111
          tunnel: [_ w245] -> _
          tunnel: w136 -> [_ w245]
          tunnel: [_ w238] -> w101
          tunnel: w99 -> [_ w237]
          tunnel: [_ w234] -> w97
          frame #0 {
            # "Add code for atten and RF switch here"
            # "Wait for RS SMT frequency to settle"
            n70 = global write "Global 2.vi" "1st Sweep"(w232) -> ()
            n71 = Wait (ms)(milliseconds to wait=10) -> ()  [unwired: 1 out]
            "1st Sweep" <- w232
          }
          frame #1 {
            # "+3.3V"
            # "Offset"
            # "Tune"
            # "Stand dev."
            # "ADCval"
            # "ACQUIRE SINGLE CHANNEL DATA\nCALCULATE MEAN AND ERROR\nSETUP FOR NEG IF VOLTAGE"
            # "# of freq steps"
            n72 = global read "Global 2.vi" "IF / LOG Det"() -> (w236:bool)
            n73 = Boolean To (0,1)(Boolean=w236) -> (0, 1=w235:i16)
            n74 = case shown="False" w236 {
              tunnel: w253 -> [w260 w261]
              tunnel: [w257 w262] -> w250
              frame False {
                n75 = Select "ADC Chan"(t=1, s=w260, f=0) -> (s? t:f=w257:i32)
              }
              frame True {
                n76 = Select "ADC Chan"(t=2, s=w261, f=3) -> (s? t:f=w262:i32)
              }
            }
            n77 = To Double Precision Float(number=w235) -> (double precision float=w234:dbl)
            n78 = global read "Global 2.vi" "# Sample/step"() -> (w242:i32)
            n79 = global read "Global 2.vi" "Tank RF"() -> (w243:bool)
            n80 = global read "Global 2.vi" "IF Atten (dB)"() -> (w241:i8)
            n81 = global read "Global 2.vi" "Logoffset (V)"() -> (w244:dbl)
            n82 = Not(x=w243) -> (.not. x?=w248:bool)
            n83 = global read "Global 2.vi" "Phase (V)"() -> (w238:dbl)
            n84 = call "Netburner_cntlTCP.vi"("Phase Volt"=w238, "Tune Volt"=w247, "# Data"=w242, "IF Atten (dB)"=w241, "NMR ADC"=w250, "Hi Gain"=w245, "Tank RF"=w248, "LogOff Volt"=w244, "IFOff Volt"=w246, "# f steps"=w249) -> ("Temp (C)"=w240:dbl, "ADC value"=w252:dbl[], "ADC Std Dev"=w251:dbl, "Volts"=w239:dbl)  [unwired: 2 out]
            "Temp (C)" <- w240
            "+3.3V supply" <- w239
            n85 = global write "Global 2.vi" "+3V supply"(w239) -> ()
            n86 = global write "Global 2.vi" "Temp (C)"(w240) -> ()
            n87 = Negate(x=w252) -> (-x=w254:dbl[])
            n88 = Wait (ms)(milliseconds to wait=1) -> ()  [unwired: 1 out]
            n89 = Select(t=w254, s=w237, f=w252) -> (s? t:f=w255:dbl[])
          }
        }
        n90 = global write "Global 2.vi" "Sweep #"(w143) -> ()
        n91 = call "Qcorrect.vi"("Subtract Q curve"=w161, "Nstep"=w71, "Max Gain"=w136, "Amp of Q curve"=w162, "Step Width (MHz)"=w117, "Center Freq (MHz)"=w118) -> ("Start"=w186:i32, "Array"=w187:dbl[])
        n92 = global read "Global 2.vi" "Real/Quad Q curve"() -> (w160:bool)
        n93 = To Double Precision Float(number=w143) -> (double precision float=w115:dbl)
        n94 = Array Subset "Array Subset"(array=w187, index=w186, length=w71) -> (w171:dbl[])
        n95 = property on="Property Node" class="VI"(reference=w91, error in=w90) -> ("Exec.State"=w93:T2)  [unwired: 2 out]
        n96 = global read "Global 2.vi" "AutoTune"() -> (w158:bool)
        n97 = Select(t=w171, s=w160, f=w169) -> (s? t:f=w84:dbl[])
        n98 = Not(x=w158) -> (.not. x?=w172:bool)
        n99 = Equal?(x=2, y=w93) -> (x = y?=→"He readback":bool)
        n100 = Not(x="Stop Run") -> (.not. x?=w88:bool)
        n101 = Greater?(x=w134, y=7.5) -> (0:w175:bool)
        n102 = Not(x=w175) -> (.not. x?=w154:bool)
        "RF OK" <- w154
        n103 = global write "Global 2.vi" "RF OK"(w154) -> ()
        n104 = global read "Global 2.vi" "Amp of Q curve"() -> (w106:dbl)
        n105 = To Double Precision Float(number=w143) -> (double precision float=w138:dbl)
        n106 = global read "Global 2.vi" "RemovePed"() -> (w159:bool)
        n107 = Equal To 0?(x=w70) -> (x = 0?=w142:bool)
        n108 = Get Date/Time In Seconds() -> (seconds since 1Jan1904=w68:timestamp)
        n109 = call "RemoveQandP.vi"("Subtract Ped?"=w159, "Qcurve"=w84, "Raw data"=w102) -> ("Ped L-R"=w180:dbl, "Corrected data"=w126:dbl[], "Ped Offfset"=w149:dbl)
        "Pedestal (V)" <- w149
        n110 = global write "Global 2.vi" "Pedestal Offset"(w149) -> ()
        n111 = global read "Global 2.vi" "Gauss Fit"() -> (w157:bool)
        n112 = global write "Global 2.vi" "Sample RMS (V)"(w119) -> ()
        n113 = global write "Global 2.vi" "Temperature (C)"(w114) -> ()
        n114 = Array Max & Min "Array Max"(array=w126) -> (max value=w110:dbl)  [unwired: 3 out]
        n115 = call-poly <vilib>:"Power Spectrum.vi"("X"=w102) -> ("Power Spectrum"=w131:dbl[])  [unwired: 1 out]
        n116 = global read "Global 2.vi" "Calib Constant"() -> (w105:dbl)
        n117 = Format Date/Time String(time format string (%c)="%c", seconds (now)=w68) -> (date/time string=→"Date / Time":string)  [unwired: 1 in]
        n118 = Absolute Value ("Abs Value")(x=w180) -> (abs(x)=w181:dbl)
        n119 = Negate(x=w180) -> (-x=w150:dbl)
        "Pedestal Diff (V)" <- w150
        n120 = call "FitData.vi"("Fit?"=w157, "Fmax"=w174, "Fmin"=w121, "Yarray"=w126) -> ("Peak Area (mV-MHz)"=w108:dbl, "Center Freq (MHz)"=w153:dbl, "NMR Graph + Fit"=w151:cluster{cluster{dbl, "Numeric":dbl}[]}[])  [unwired: 2 out]
        "Peak area (V-MHz)" <- w108
        "Peak center (MHz)" <- w153
        n121 = Build Array (concatenate) "Header + Data"(w118, w117, w116, w115, w114, w113, w112, w111, w101, w108, w106, w105, w103, w98, w97, w102) -> (w132:dbl[])
        n122 = global write "Global 2.vi" "Peak area (mV-MHz)"(w108) -> ()
        n123 = Square Root(x=w131) -> (sqrt(x)=w127:dbl[])
        "FFT Vrms" <- w127
        n124 = global write "Global 2.vi" "NMR Graph + Fit"(w151) -> ()
        n125 = call "SaveData.vi"("Array"=w132, "Save Data to File"=TRUE, "Ext time (sec)"=w177) -> ()  [unwired: 1 out]
        n126 = global write "Global 2.vi" "Pedestal Difference"(w150) -> ()
        n127 = global write "Global 2.vi" "Pedestal Diff (V)"(w150) -> ()
        n128 = Select(t=w102, s=w123, f=w127) -> (s? t:f=w82:dbl[])
        n129 = feedback #2 "Feedback Node"() -> (w141:dbl[])  [unwired: 1 in]
        n130 = case shown="False" w142 {
          tunnel: w82 -> [w213 w215]
          tunnel: [w212 w215] -> w139
          tunnel: w141 -> [w214 _]
          frame False {
            # "Sum sweeps"
            n131 = Add(x=w214, y=w213) -> (x+y=w212:dbl[])
          }
          frame True {
            # "Initialize"
          }
        }
        n132 = feedback-in #2(w139) -> ()
        n133 = Divide(x=w139, y=w138) -> (x/y=w83:dbl[])
        n134 = Multiply(x=w105, y=w110) -> (x*y=w109:dbl)
        n135 = Select(t=0.1, s=w136, f=0.01) -> (s? t:f=w144:dbl)
        n136 = Multiply(x=w108, y=w105) -> (x*y=w107:dbl)
        n137 = Greater?(x=w181, y=w144) -> (0:w146:bool)
        n138 = call "ADCok.vi"("PedOK"=w146, "Array"=w102, "Vmax-1/2"=w140) -> ("Vmin"=w166:dbl, "ADC voltages OK"=w156:bool, "Allok"=w173:bool)
        "ADC volts OK" <- w156
        n139 = Multiply(x=w166, y=10.0) -> (x*y=w164:dbl)
        n140 = call "Autozero.vi"("Vmin (V)"=w164, "IFoffset (V)"=w134, "Enable"=w172, "Max Gain"=w136) -> ()
        n141 = global read "Global - Pressure & Flow.vi" "Task3 Temperature"() -> (→"He temp (K)":dbl)
        n142 = global read "Global - Pressure & Flow.vi" "Task3 Pressure"() -> (→"He press (torr)":dbl)
        n143 = And(x=w173, y=w145) -> (x .and. y?=w182:bool)
        n144 = case shown="False" w173 {
          frame False {
            # "All OK"
            n145 = property on="Raw NMR Graph / Ave" class="WFGraph (strict)"("Active Plot"=0, "Plot.Plot Color"=u32 13145856) -> ()  [unwired: 2 in, 2 out]
          }
          frame True {
            # "Bad data"
            n146 = property on="Raw NMR Graph / Ave" class="WFGraph (strict)"("Active Plot"=0, "Plot.Plot Color"=u32 16711680) -> ()  [unwired: 2 in, 2 out]
          }
        }
        n147 = Not(x=w146) -> (.not. x?=w155:bool)
        "Pedestal OK" <- w155
        n148 = global write "Global 2.vi" "Peak center (MHz)"(w153) -> ()
        n149 = Select(t=w107, s=w157, f=w109) -> (s? t:f=w152:dbl)
        "Peak amp (V)" <- w152
        n150 = global read "Global 2.vi" "Subtract Q curve"() -> (w85:bool)
        n151 = case shown="False" w85 {
          tunnel: w82 -> [w207 w211]
          tunnel: [w206 w210] -> w86
          tunnel: w84 -> [_ w209]
          tunnel: w69 -> [w205 w208]
          frame False {
            n152 = Build Array(w207, w205) -> (w206:dbl[][])
          }
          frame True {
            n153 = Build Array(w211, w208, w209) -> (w210:dbl[][])
          }
        }
        n154 = Select(t=w121, s=w123, f=0.0) -> (s? t:f=w120:dbl)
        n155 = Select(t=w117, s=w123, f=1.0) -> (s? t:f=w124:dbl)
        n156 = global write "Global 2.vi" "Pedestal OK"(w155) -> ()
        n157 = global write "Global 2.vi" "ADC volts OK"(w156) -> ()
        n158 = case shown="True" w182 {
          tunnel: [w220 -99.0] -> w183
          tunnel: w152 -> [w220 _]
          frame False {
            # "Data OK"
          }
          frame True {
            # "flag it bad"
          }
        }
        n159 = global write "Global 2.vi" "Peak Height"(w152) -> ()
        n160 = global write "Global 2.vi" "Peak amp (V)"(w152) -> ()
        n161 = Bundle(w120, "Step Width (MHz)"=w124, w86) -> (→"Raw NMR Graph / Ave":cluster{dbl, "Step Width (MHz)":dbl, dbl[][]})  [unwired: 1 in]
        n162 = Build Array (concatenate) "Build Array"(w120, w124, w83) -> (w135:dbl[])
      }
      n163 = call "DataQA.vi"("Quality cuts"=w54, "Data In"=w62) -> ("Data Out"=w61:dbl[])
      n164 = global read "Global 2.vi" "Save Data to File"() -> (w47:bool)
      n165 = call <vilib>:"Std Deviation and Variance.vi"("X"=w61) -> ("mean"=w52:dbl, "standard deviation"=w42:dbl)  [unwired: 1 in, 1 out]
      "Peak mean (V)" <- w52
      n166 = Multiply(x=w42, y=1000.0) -> (x*y=→"Peak RMS (mV)":dbl)
      n167 = call "PeakHisto.vi"("Data Out"=w61) -> ("XY Graph"=w50:cluster{"Y":dbl[], "Y":dbl[]}[])
      "Peak Height Distribution" <- w50
      n168 = global write "Global 2.vi" "Peak Height Distribution"(w50) -> ()
      n169 = global write "Global 2.vi" "Peak mean (V)"(w52) -> ()
      n170 = call "SaveDataAve.vi"("Array"=w48, "Save Data to File"=w47) -> ()  [unwired: 1 in, 1 out]
      n171 = Array Size(array=w61) -> (size(s)=w51:i32)
      "# Good Spectra" <- w51
      n172 = global write "Global 2.vi" "# Good Spectra"(w51) -> ()
      n173 = Divide(x=w52, y=w42) -> (x/y=w53:dbl)
      "S/N" <- w53
      n174 = global write "Global 2.vi" "S/N"(w53) -> ()
    }
    frame #2 {
      n175 = property on="Property Node" class="VI"(reference=w266, error in=w265) -> (reference out=w268:refnum<vi>, error out=w267:errorcluster, "Exec.State"=w270:T2)
      n176 = Equal?(x=2, y=w270) -> (x = y?=w269:bool)
      n177 = case shown="True" w269 {
        tunnel: w268 -> [_ w277]
        tunnel: w267 -> [_ w276]
        frame False {
        }
        frame True {
          # "Stop MKS routine and close panel if running"
          # "Add simple error handling\nfor VI operations"
          n178 = invoke on="Invoke Node" class="VI" method="Abort VI"(reference=w277, error in=w276) -> (reference out=w274:refnum<vi>, error out=w273:errorcluster)  [unwired: 1 in, 1 out]
          n179 = property on="Property Node" class="VI"(reference=w274, error in=w273, "Front Panel Window:Open"=FALSE) -> (error out=w272:errorcluster)  [unwired: 1 out]
          n180 = call <vilib>:"Simple Error Handler.vi"("type of dialog (OK msg:1)"=1, "error in (no error)"=w272) -> ()  [unwired: 3 in, 5 out]
        }
      }
    }
  }
